vi "AddAdditionalFields.vi"(8 "error in (no error)":errorcluster, 10 "Menu":refnum<class "MGI_Menu.lvclass">, 11 "MenuItem in":refnum<class "MGI_ToolStripItem.lvclass">) -> (0 "error out":errorcluster, 2 "Menu out":refnum<class "MGI_Menu.lvclass">, 3 "MenuItem out":refnum<class "MGI_ToolStripItem.lvclass">)   [LabVIEW 2019, in "MGI_ToolStripItem.lvclass"]
doc: "No-op for a standard Menu Item. Used by children classes to add additional fields (Like shortcuts, etc)\n\nAuthored by Derek E. Trepanier\nsupport@mooregoodideas.com\nwww.mooregoodideas.com\n\nCopyright (c) 2012, Moore Good Ideas, Inc.\n\nAll rights reserved.\n\nRedistribution and use in source and binary forms, with or without modification, are permitted provided that the following conditions are met:\n\n * Redistributions of source code must retain the above copyright notice, this list of conditions and the following disclaimer.\n * Redistributions in binary form must reproduce the above copyright notice, this list of conditions and the following disclaimer in the documentation and/or other materials provided with the distribution.\n * Neither the name of Moore Good Ideas, Inc. nor the names of its contributors may be used to endorse or promote products derived from this software without specific prior written permission.\n\nTHIS SOFTWARE IS PROVIDED BY THE COPYRIGHT HOLDERS AND CONTRIBUTORS \"AS IS\" AND ANY EXPRESS OR IMPLIED WARRANTIES, INCLUDING, BUT NOT LIMITED TO, THE IMPLIED WARRANTIES OF MERCHANTABILITY AND FITNESS FOR A PARTICULAR PURPOSE ARE DISCLAIMED. IN NO EVENT SHALL THE COPYRIGHT OWNER OR CONTRIBUTORS BE LIABLE FOR ANY DIRECT, INDIRECT, INCIDENTAL, SPECIAL, EXEMPLARY, OR CONSEQUENTIAL DAMAGES (INCLUDING, BUT NOT LIMITED TO, PROCUREMENT OF SUBSTITUTE GOODS OR SERVICES; LOSS OF USE, DATA, OR PROFITS; OR BUSINESS INTERRUPTION) HOWEVER CAUSED AND ON ANY THEORY OF LIABILITY, WHETHER IN CONTRACT, STRICT LIABILITY, OR TORT (INCLUDING NEGLIGENCE OR OTHERWISE) ARISING IN ANY WAY OUT OF THE USE OF THIS SOFTWARE, EVEN IF ADVISED OF THE POSSIBILITY OF SUCH DAMAGE."
uses:
  MGI_ToolStripItem.lvclass
  C:/Program Files (x86)/National Instruments/LabVIEW 2019/user.lib/_MGI/Menu Building/MenuItem/MGI_MenuItem.lvclass
  <userlib>/_MGI/Menu Building/MenuTypes/MGI_Menu.lvclass
  ToolStrip/MGI_ToolStrip.lvclass
  C:/Program Files (x86)/National Instruments/LabVIEW 2019/user.lib/_MGI/Menu Building/MenuTypes/MGI_Menu.lvclass
  MGI_ToolStripItem.lvclass/MGI_ToolStripItem.ctl
  System.Drawing
  System.Windows.Forms
  <userlib>/_MGI/Menu Building/MenuItem/Read Full Tag.vi
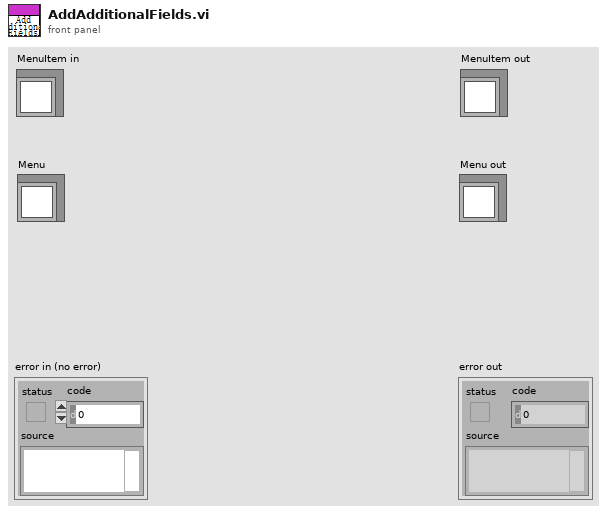
[diagram p1: front panel]
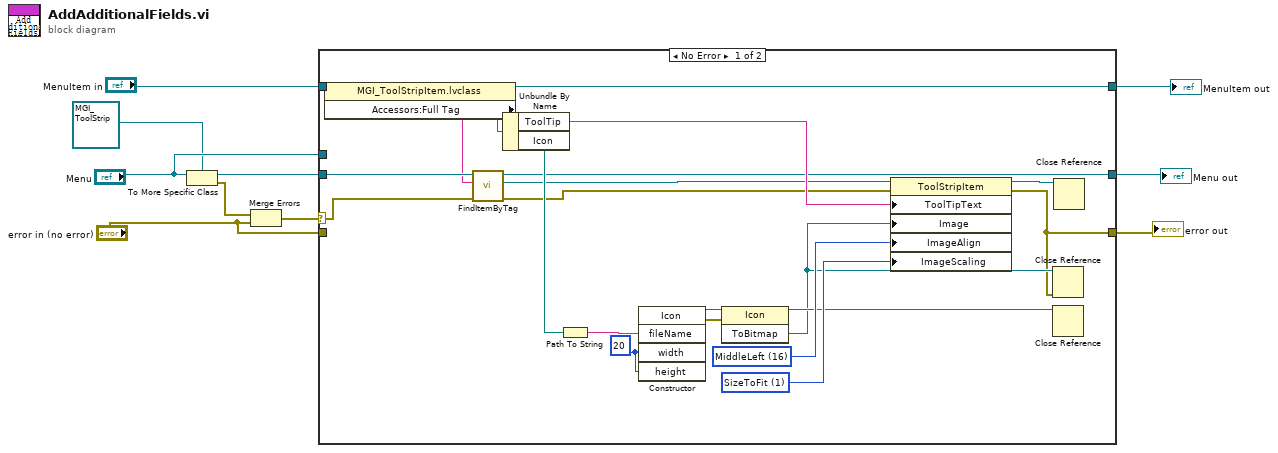
[diagram p0: block diagram]
diagram:
  n1 = To More Specific Class(target class=refnum<class "MGI_ToolStrip.lvclass"> refnum ("MGI_ToolStrip.lvclass"), reference="Menu") -> (specific class reference=w10:refnum<class "MGI_ToolStrip.lvclass">, error out=w8:errorcluster)  [unwired: 1 in]
  n2 = Merge Errors(w8, "error in (no error)") -> (w9:errorcluster)
  n3 = case shown="No Error" w9 {
    selector: w9 -> [w14 _]
    tunnel: [w17 w32] -> w4
    tunnel: [w11 w31] -> w5
    tunnel: w10 -> [w16 _]
    tunnel: [w29 w33] -> w6
    tunnel: "MenuItem in" -> [w30 w33]
    tunnel: "error in (no error)" -> [_ w32]
    tunnel: "Menu" -> [_ w31]
    frame No Error {
      w23 = 1 items=["None", "SizeToFit"] ("ImageScaling")
      w24 = 16 items=["TopLeft"=1, "TopCenter"=2, "TopRight"=4, "MiddleLeft"=16, "MiddleCenter"=32, "MiddleRight"=64, "BottomLeft"=256, "BottomCenter"=512, "BottomRight"=1024] ("ImageAlign")
      w27 = 20 ("width")
      n4 = property class="MGI_ToolStripItem.lvclass"(reference=w30) -> (reference out=w29:refnum<class "MGI_ToolStripItem.lvclass">, "Accessors:Full Tag"=w15:string)  [unwired: 1 in, 1 out]
      n5 = call "FindItemByTag.vi"("error in (no error)"=w14, "Tag"=w15, "MGI_ToolStrip in"=w16) -> ("error out"=w13:errorcluster, "ToolStripItem"=w12:refnum<k24>, "MGI_ToolStrip out"=w11:refnum<class "MGI_ToolStrip.lvclass">)  [unwired: 6 in]
      n6 = Unbundle By Name(w29) -> ("ToolTip"=w28:string, "Icon"=w22:path)
      n7 = Path To String(path=w22) -> (string=w21:string)
      n8 = constructor class="Icon"("fileName"=w21, "width"=w27, "height"=w27) -> (reference out=w25:refnum<k24>, error out=w26:errorcluster)  [unwired: 3 in, 4 out]
      n9 = invoke class="Icon" method="ToBitmap"(reference=w25, error in=w26) -> (reference out=w19:refnum<k24>, "ToBitmap"=w18:refnum<k24>)  [unwired: 1 in, 1 out]
      n10 = property class="ToolStripItem"(reference=w12, error in=w13, "ToolTipText"=w28, "Image"=w18, "ImageAlign"=w24, "ImageScaling"=w23) -> (reference out=w20:refnum<k24>, error out=w17:errorcluster)
      n11 = Close Reference(reference=w18, error in (no error)=w17) -> ()  [unwired: 1 out]
      n12 = Close Reference(reference=w19) -> ()  [unwired: 1 in, 1 out]
      n13 = Close Reference(reference=w20) -> ()  [unwired: 1 in, 1 out]
    }
    frame Error {
    }
  }
  "error out" <- w4
  "MenuItem out" <- w6
  "Menu out" <- w5
